vi "Log event.vi"(8 "error in (no error)":errorcluster, 10 "Data in":variant, 11 "Logger in":refnum<class "Logger.lvclass">) -> (0 "error out":errorcluster, 2 "Data out":variant, 3 "Logger out":refnum<class "Logger.lvclass">)   [LabVIEW 2020, in "Module.lvlib" / "Logger.lvclass"]
uses:
  Logger.lvclass
panel:
  in  "Class":string(combo)
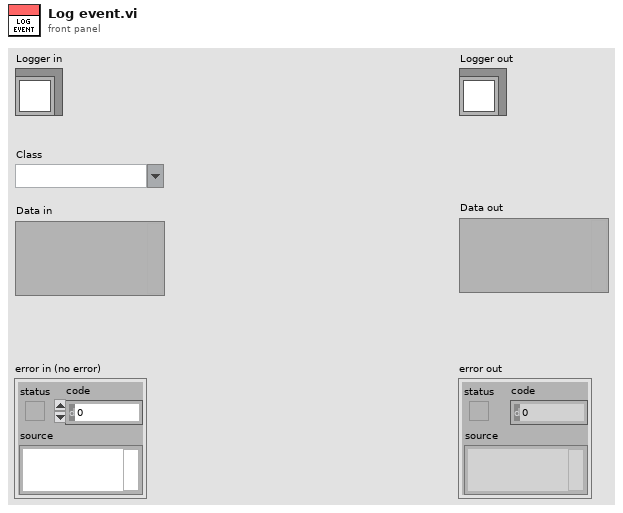
[diagram p1: front panel]
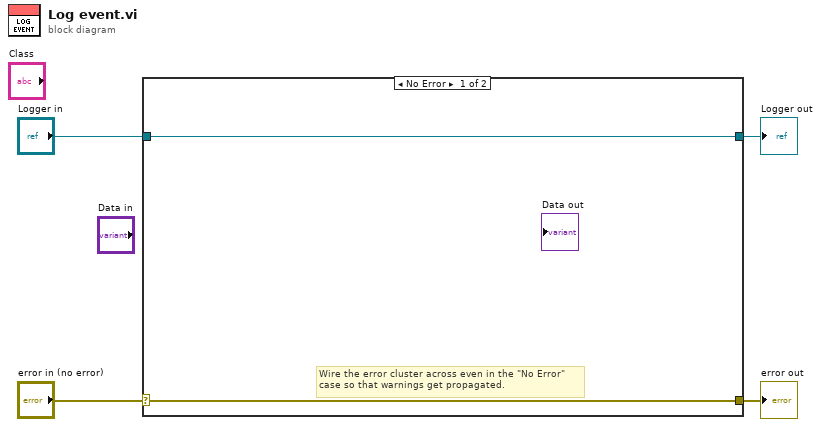
[diagram p0: block diagram]
diagram:
  n1 = case shown="No Error" "error in (no error)" {
    selector: "error in (no error)" -> [w5 w8]
    tunnel: [w5 w8] -> w3
    tunnel: [w6 w7] -> w1
    tunnel: "Logger in" -> [w6 w7]
    frame No Error {
      # "Wire the error cluster across even in the \"No Error\"\ncase so that warnings get propagated."
    }
    frame Error {
    }
  }
  "error out" <- w3
  "Logger out" <- w1
